vi "FMA1600A Raw Serial Read Write.vi"(8 "error in (no error)":errorcluster, 10 "String":string, 11 "VISA Refnum in":refnum<visa-resource-name>) -> (0 "error out":errorcluster, 2 "Data Stream":string, 3 "VISA Refnum out":refnum<visa-resource-name>)   [LabVIEW 2020]
panel:
  out "Serial Settings:Number of Bytes at Serial Port":u32
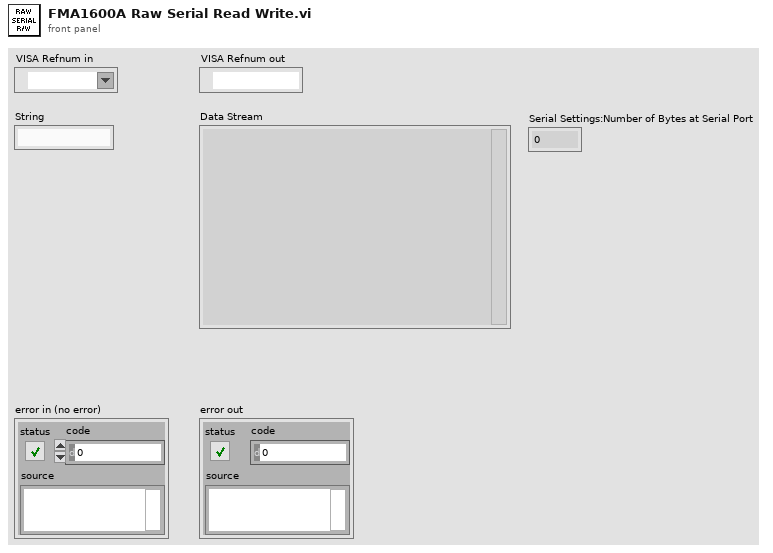
[diagram p1: front panel]
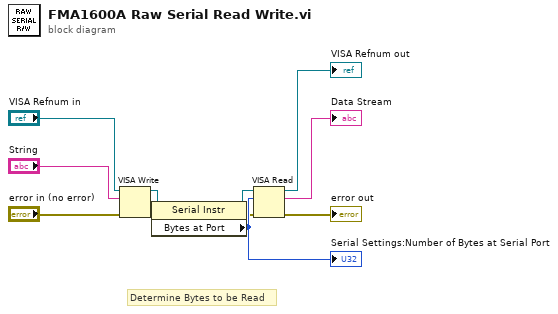
[diagram p0: block diagram]
diagram:
  # "Determine Bytes to be Read"
  n1 = VISA Write(VISA resource name="VISA Refnum in", write buffer="String", error in (no error)="error in (no error)") -> (VISA resource name out=w7:refnum<visa-resource-name>, error out=w9:errorcluster)  [unwired: 1 out]
  n2 = property class="Serial Instr"(reference=w7, error in=w9) -> (reference out=w8:refnum<visa-resource-name>, error out=w10:errorcluster, "Bytes at Port"=w11:u32)
  "Serial Settings:Number of Bytes at Serial Port" <- w11
  n3 = VISA Read(VISA resource name=w8, byte count=w11, error in (no error)=w10) -> (VISA resource name out=→"VISA Refnum out":refnum<visa-resource-name>, read buffer=→"Data Stream":string, error out=→"error out":errorcluster)  [unwired: 1 out]
